vi "AwaitDriverError.vi"(8 "error in (no error)":errorcluster, 10 "status":i32, 11 "Occurrence in":refnum<k4>) -> (0 "error out":errorcluster)   [LabVIEW 2020, in "NI_TargetHelper.lvlib"]
uses:
  <vilib>/TargetSupport/NI_TargetHelper/NI_TargetHelper.lvlib
  <vilib>/rvi/interface/common/niFpgaWaitOnOcc.vi
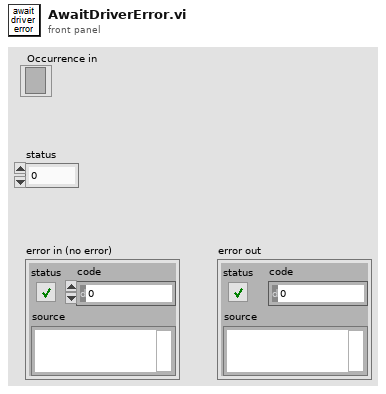
[diagram p1: front panel]
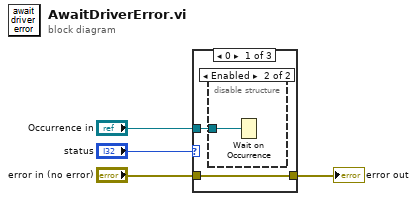
[diagram p0: block diagram]
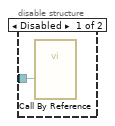
[diagram p2: hidden frame]
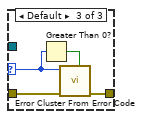
[diagram p4: hidden frame]
diagram:
  n1 = case shown="0" "status" {
    selector: "status" -> [_ _ w10]
    tunnel: [w6 w9 w12] -> w4
    tunnel: "error in (no error)" -> [w6 w9 w13]
    tunnel: "Occurrence in" -> [w5 _ _]
    frame 0 {
      n2 = disable-structure shown="Enabled" {
        disable-tunnel: w5 -> [w7 w8]
        frame Disabled {
          n3 = call-by-ref "?"("occurrence"=w7) -> ()  [unwired: 16 in, 3 out]
        }
        frame Enabled {
          n4 = Wait on Occurrence(2:w8) -> ()  [unwired: 2 in, 1 out]
        }
      }
    }
    frame -61167 {
      # "emulation case intentionally ignoring error"
    }
    frame Default {
      n5 = Greater Than 0?(x=w10) -> (x > 0?=w11:bool)
      n6 = call <vilib>:"Error Cluster From Error Code.vi"("is warning? (False)"=w11, "error in (no error)"=w13, "error code (0)"=w10) -> ("error out"=w12:errorcluster)  [unwired: 6 in]
    }
  }
  "error out" <- w4
